vi "New File from Path.vi"(8 "error in (no error)":errorcluster, 10 "Path":path) -> (0 "error out":errorcluster, 3 "File out":refnum<class "File.lvclass">)   [LabVIEW 2020, in "Save for Previous Version.lvlib" / "File.lvclass"]
uses:
  File.lvclass
  File.lvclass/File.ctl
  Write Path.vi
  Write is LabVIEW File Type.vi
  LabVIEW File/LabVIEW File.lvclass
  \\Mac\Home/JKI/GitHub/vipm-io/a-version-explorer-for-labview/experiments/save-for-previous-version/source/File/File.lvclass/File.lvclass
  <vilib>/Utility/lvfile.llb/NI_FileType.lvlib
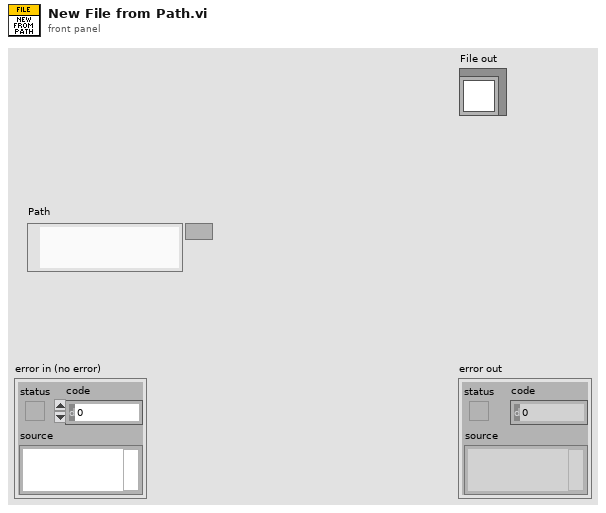
[diagram p1: front panel]
types:
  T1 = typedef "NI_FileType.lvlib/FT_FileTypes.ctl" = enum32{"Invalid file/path", "Unknown type", "Instrument", "Control", "Polymorphic VI", "Project", "Library", "LVClass", "XControl", "XNode", "CIN", "Run-time menu", "Palette menu", "LLB", "Shortcut", "Directory", "Class Private Data Control", "Statechart", "MathScript .m file", "Ladder Diagram", "LVLibp"}
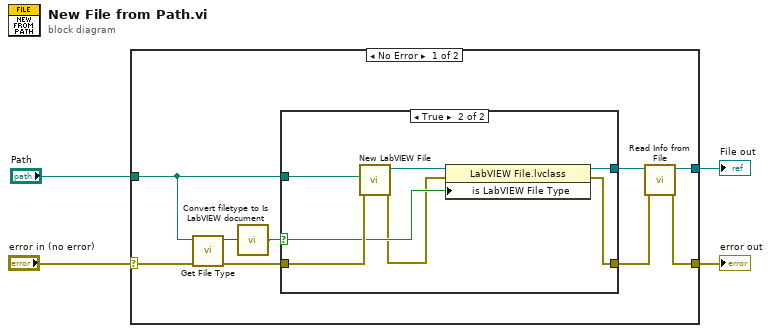
[diagram p0: block diagram]
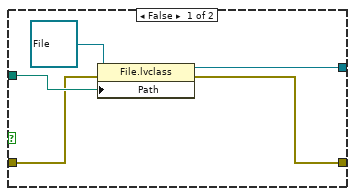
[diagram p2: hidden frame]
diagram:
  n1 = case shown="No Error" "error in (no error)" {
    selector: "error in (no error)" -> [w10 w26]
    tunnel: [w5 w26] -> w3
    tunnel: [w7 _] -> w2
    tunnel: "Path" -> [w11 _]
    frame No Error {
      n2 = call <vilib>:"Get File Type.vi"("error in (no error)"=w10, "path"=w11) -> ("error out"=w9:errorcluster, "file type"=w13:T1)  [unwired: 7 in, 1 out]
      n3 = call <vilib>:"Convert filetype to Is LabVIEW document.vi"("file type"=w13) -> ("Is LabVIEW document?"=w12:bool)  [unwired: 4 in]
      n4 = case shown="True" w12 {
        selector: w12 -> [_ w21]
        tunnel: w11 -> [w18 w23]
        tunnel: [w17 w22] -> w8
        tunnel: [w16 w19] -> w6
        tunnel: w9 -> [w15 w24]
        frame False {
          n5 = property class="File.lvclass"(reference=refnum<class "File.lvclass"> refnum, error in=w15, "Path"=w18) -> (reference out=w17:refnum<class "File.lvclass">, error out=w16:errorcluster)
        }
        frame True {
          n6 = call "New LabVIEW File.vi"("error in (no error)"=w24, "Path"=w23) -> ("error out"=w20:errorcluster, "LabVIEW File out"=w25:refnum<class "LabVIEW File.lvclass">)  [unwired: 8 in]
          n7 = property class="LabVIEW File.lvclass"(reference=w25, error in=w20, "is LabVIEW File Type"=w21) -> (reference out=w22:refnum<class "LabVIEW File.lvclass">, error out=w19:errorcluster)
        }
      }
      n8 = call-dynamic "Read Info from File.vi"("error in (no error)"=w6, "File in"=w8) -> ("error out"=w5:errorcluster, "File out"=w7:refnum<class "File.lvclass">)  [unwired: 8 in]
    }
    frame Error {
    }
  }
  "error out" <- w3
  "File out" <- w2
